vi "LED_MODE - Type.vi"(8 "error in (no error)":errorcluster, 11 "LED_MODE":T1) -> (0 "error out":errorcluster, 3 "LED_MODE_VALUE":i32)   [LabVIEW 2013]
doc: "<b>Camera LED state options.</b>\nHEARTBEAT : Blink if link is ok (led 1), heartbeat mode (led 2).\nTRIGGER_ACTIVE : Blink led if trigger detected.\nEXT_EVENT_ACTIVE : Blink led if external signal detected.\nACQUISITION : Blink led during data streaming.\nEXPOSURE_ACTIVE : Blink led during sensor integration time.\nFRAME_ACTIVE : Blink if device busy/not busy.\nLINK : Blink led if link is ok.\nOFF : Set led to zero.\nON : Set led to one."
uses:
  LED_MODE.ctl
  C:/Projects/Cameras3.x/xiLib/xiLIB_64bit/xiLIB/xiCamLib/API/x64/xiApi.NETX64.dll
  xiLIB_64bit/xiLIB/xiCamLib/API/x64/xiApi.NETX64.dll
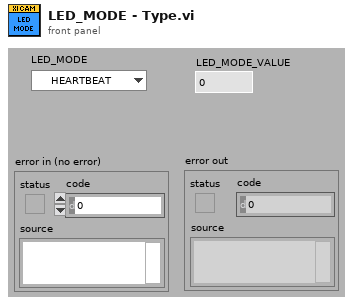
[diagram p1: front panel]
types:
  T1 = typedef "LED_MODE.ctl" = enum16{"HEARTBEAT", "TRIGGER_ACTIVE", "EXT_EVENT_ACTIVE", "ACQUSITION", "EXPOSURE_ACTIVE", "FRAME_ACTIVE", "LINK", "OFF", "ON"}
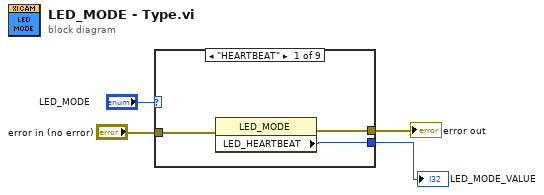
[diagram p0: block diagram]
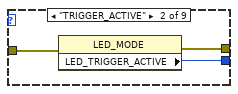
[diagram p2: hidden frame]
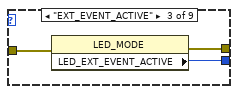
[diagram p3: hidden frame]
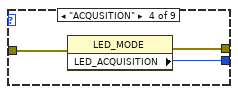
[diagram p4: hidden frame]
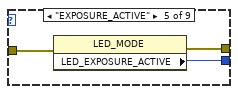
[diagram p5: hidden frame]
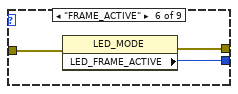
[diagram p6: hidden frame]
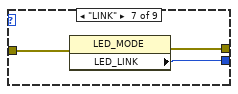
[diagram p7: hidden frame]
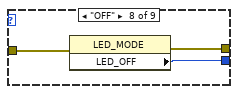
[diagram p8: hidden frame]
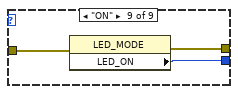
[diagram p9: hidden frame]
diagram:
  n1 = case shown="\"HEARTBEAT\"" "LED_MODE" {
    tunnel: "error in (no error)" -> [w7 w10 w13 w16 w19 w22 w25 w28 w31]
    tunnel: [w6 w9 w12 w15 w18 w21 w24 w27 w30] -> w2
    tunnel: [w5 w8 w11 w14 w17 w20 w23 w26 w29] -> w1
    frame "HEARTBEAT" {
      n2 = property class="LED_MODE"(error in=w7) -> (error out=w6:errorcluster, "LED_HEARTBEAT"=w5:i32)  [unwired: 1 in, 1 out]
    }
    frame "TRIGGER_ACTIVE" {
      n3 = property class="LED_MODE"(error in=w10) -> (error out=w9:errorcluster, "LED_TRIGGER_ACTIVE"=w8:i32)  [unwired: 1 in, 1 out]
    }
    frame "EXT_EVENT_ACTIVE" {
      n4 = property class="LED_MODE"(error in=w13) -> (error out=w12:errorcluster, "LED_EXT_EVENT_ACTIVE"=w11:i32)  [unwired: 1 in, 1 out]
    }
    frame "ACQUSITION" {
      n5 = property class="LED_MODE"(error in=w16) -> (error out=w15:errorcluster, "LED_ACQUISITION"=w14:i32)  [unwired: 1 in, 1 out]
    }
    frame "EXPOSURE_ACTIVE" {
      n6 = property class="LED_MODE"(error in=w19) -> (error out=w18:errorcluster, "LED_EXPOSURE_ACTIVE"=w17:i32)  [unwired: 1 in, 1 out]
    }
    frame "FRAME_ACTIVE" {
      n7 = property class="LED_MODE"(error in=w22) -> (error out=w21:errorcluster, "LED_FRAME_ACTIVE"=w20:i32)  [unwired: 1 in, 1 out]
    }
    frame "LINK" {
      n8 = property class="LED_MODE"(error in=w25) -> (error out=w24:errorcluster, "LED_LINK"=w23:i32)  [unwired: 1 in, 1 out]
    }
    frame "OFF" {
      n9 = property class="LED_MODE"(error in=w28) -> (error out=w27:errorcluster, "LED_OFF"=w26:i32)  [unwired: 1 in, 1 out]
    }
    frame "ON" {
      n10 = property class="LED_MODE"(error in=w31) -> (error out=w30:errorcluster, "LED_ON"=w29:i32)  [unwired: 1 in, 1 out]
    }
  }
  "error out" <- w2
  "LED_MODE_VALUE" <- w1
